vi "Anna_Auto.vi"() -> ()   [LabVIEW 2009]
panel:
  in  "notes":string
  out "Int duplex?":bool
  out "TACwinLoaded?":bool
  out "16btimage?":bool
  out "router":u8(ring) items=["sum", "0", "1", "2", "3", "4", "5", "6", "7", "8", "9", "10", "11", "12", "13", "14", "15"]
  out "plane":u32
  in  "router channel":u8
  in  "Value":cluster{"max":u32, "min":u32}
  out "what is done?":string
  in  "Folder Path":path
  out "what file?":path
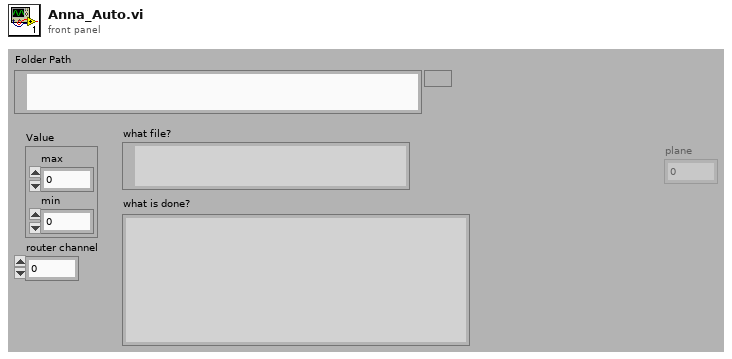
[diagram p1: front panel]
types:
  T1 = enum16{"Get", "Set", "Change", "ini", "clear", "draw", "draw false"}
  T2 = enum32{"existing file", "new file", "new or existing file", "existing dir", "new dir", "new or existing dir", "existing file (use LLBs)", "new file (use LLBs)", "new or existing file (use LLBs)", "new or existing file or directory (use LLBs)"}
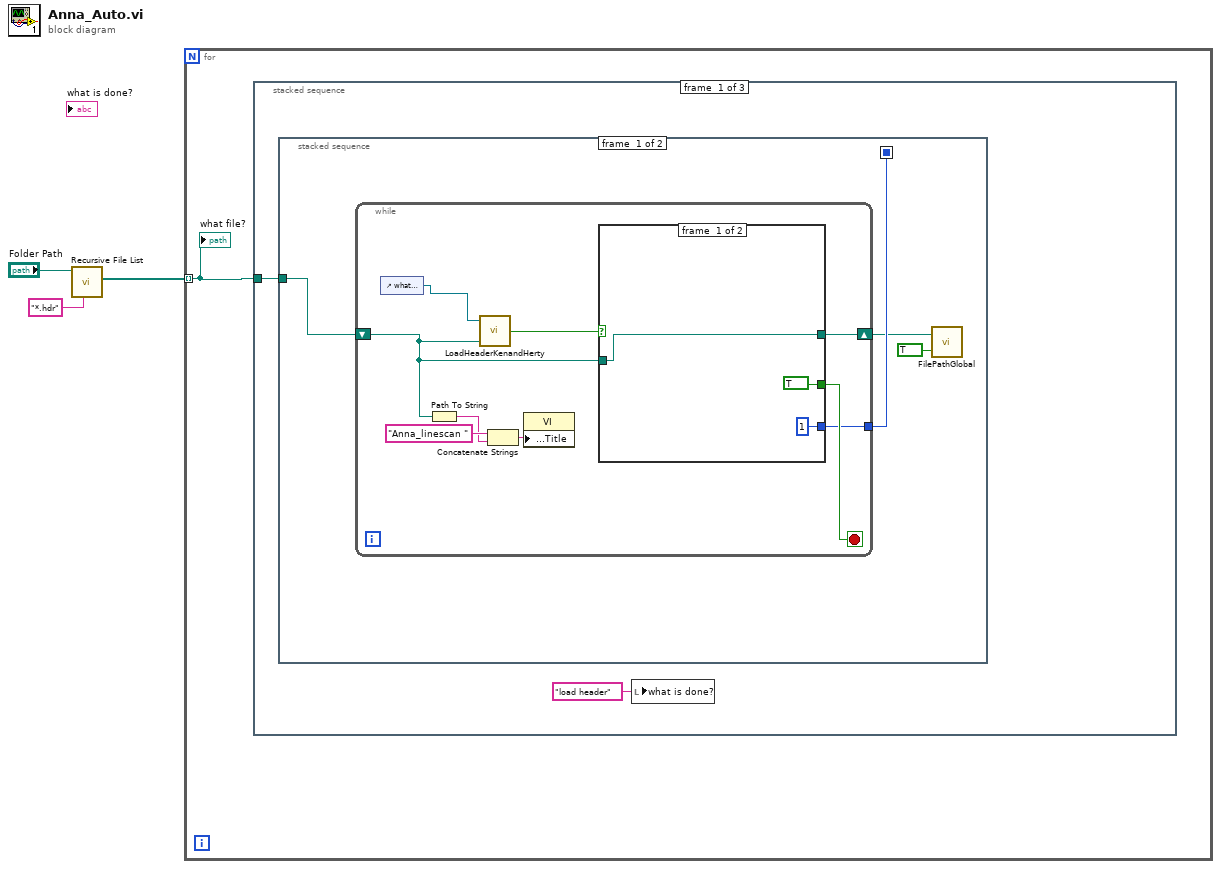
[diagram p0: block diagram]
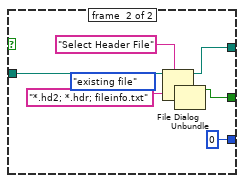
[diagram p2: hidden frame]
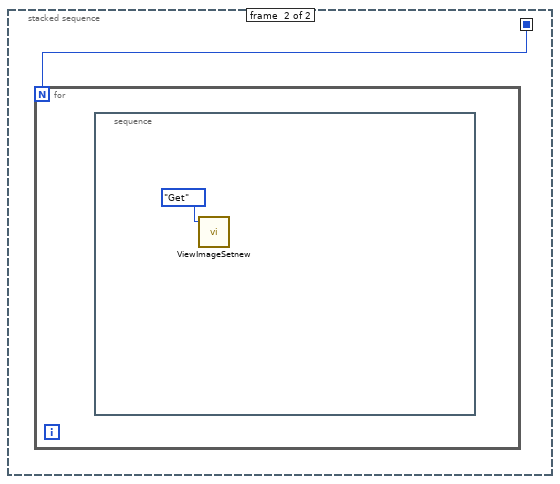
[diagram p3: hidden frame]
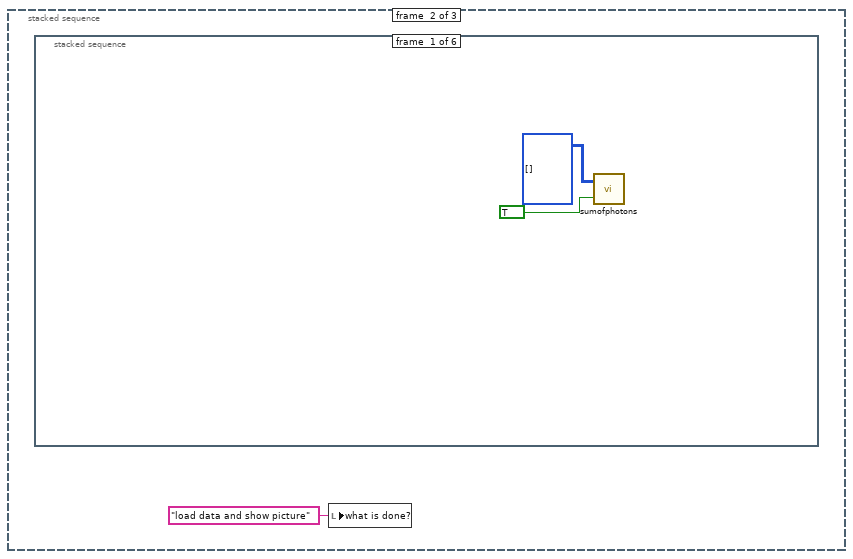
[diagram p4: hidden frame]
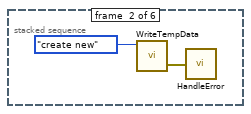
[diagram p5: hidden frame]
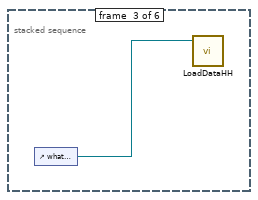
[diagram p6: hidden frame]
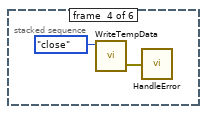
[diagram p7: hidden frame]
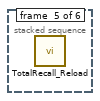
[diagram p8: hidden frame]
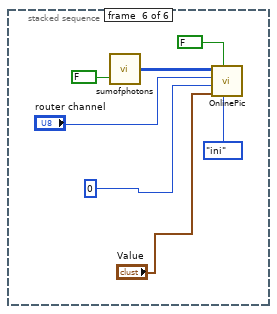
[diagram p9: hidden frame]
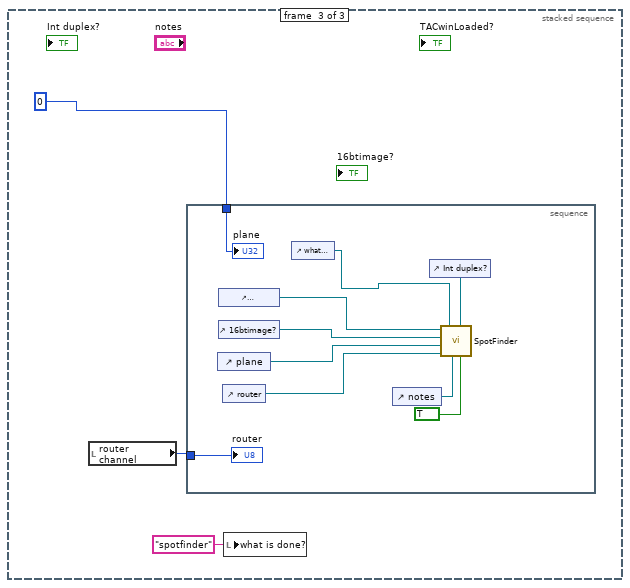
[diagram p10: hidden frame]
diagram:
  n1 = call <vilib>:"Recursive File List.vi"("pattern"="*.hdr", "Folder Path"="Folder Path") -> ("All Files in Dir"=w3:path[])  [unwired: 5 in, 4 out]
  n2 = for {
    tunnel: w3 -> [w4] mode=indexing
    n3 = stacked-sequence {
      tunnel: w4 -> [w6 _ _]
      frame #0 {
        n4 = stacked-sequence {
          seq-local: [w10 _] -> [_ w30]
          tunnel: w6 -> [w7 _]
          frame #0 {
            n5 = while {
              shift-right: [w13] -> w9
              shift-left: w7 -> [w14]
              tunnel: [w12] -> w10
              stop <- w15 stop-if-true
              n6 = control-ref of="what file?"() -> (w11:refnum<vi>)
              n7 = Path To String(path=w14) -> (string=w17:string)
              n8 = call "LoadHeaderKenandHerty.vi"("appended path"=w14, "reference"=w11) -> ("unsuccesful?"=w16:bool)  [unwired: 3 in]
              n9 = Concatenate Strings("Anna_linescan " ("string"), w17) -> (w19:string)
              n10 = property class="VI"("Front Panel Window:Title"=w19) -> ()  [unwired: 2 in, 2 out]
              n11 = case shown="False" w16 {
                tunnel: w14 -> [w20 w29]
                tunnel: [TRUE w25] -> w15
                tunnel: [w20 w27] -> w13
                tunnel: [1 0] -> w12
                frame #0 {
                }
                frame #1 {
                  (unwired) T2."existing file" ("select mode (2)")
                  n12 = File Dialog(6:"*.hd2; *.hdr; fileinfo.txt" ("pattern"), 7:"Select Header File" ("prompt"), 11:w29) -> (0:w23:errorcluster, 1:w25:bool, 3:w27:path)  [unwired: 4 in, 1 out]
                  n13 = Unbundle(w23) -> ()  [unwired: 3 out]
                }
              }
            }
            n14 = call "FilePathGlobal.vi"("Image Path"=w9, "set?"=TRUE) -> ()  [unwired: 3 out]
          }
          frame #1 {
            n15 = for {
              N: w30 -> [_]
              n16 = stacked-sequence {
                frame #0 {
                  n17 = call "ViewImageSetnew.vi"("action"=enum16{"Display", "change", "Get", "Set"}."Get" ("Enum")) -> ()  [unwired: 2 in, 1 out]
                }
              }
            }
          }
        }
        n18 = local write "what is done?"("load header" ("what is done?")) -> ()
      }
      frame #1 {
        n19 = stacked-sequence {
          frame #0 {
            n20 = call "sumofphotons.vi"("s"=TRUE, "sum of photons"=u32[][][][] []) -> ()  [unwired: 1 out]
          }
          frame #1 {
            n21 = call "WriteTempData.vi"("Enum"=enum16{"create new", "write", "close"}."create new") -> ("error out"=w35:errorcluster)  [unwired: 4 in, 1 out]
            n22 = call "HandleError.vi"("error in (no error)"=w35) -> ()
          }
          frame #2 {
            n23 = control-ref of="what file?"() -> (w37:refnum<vi>)
            n24 = call "LoadDataHH.vi"("Path"=w37) -> ()  [unwired: 2 in, 3 out]
          }
          frame #3 {
            n25 = call "WriteTempData.vi"("Enum"=enum16{"create new", "write", "close"}."close") -> ("error out"=w38:errorcluster)  [unwired: 4 in, 1 out]
            n26 = call "HandleError.vi"("error in (no error)"=w38) -> ()
          }
          frame #4 {
            n27 = call "TotalRecall_Reload.vi"() -> ()  [unwired: 4 in, 4 out]
          }
          frame #5 {
            n28 = call "sumofphotons.vi"("s"=FALSE) -> ("sum of photons out"=w44:u32[][][][])  [unwired: 1 in]
            n29 = call "OnlinePic.vi"("action"=T1."ini" ("Enum"), "RGB/False"=FALSE, "Threshold (max)"="Value", "plane"=u32 0, "router channel"="router channel", "Array"=w44) -> ()  [unwired: 1 in, 5 out]
          }
        }
        n30 = local write "what is done?"("load data and show picture" ("what is done?")) -> ()
      }
      frame #2 {
        n31 = local read "router channel"() -> (w47:u8)
        n32 = stacked-sequence {
          tunnel: u32 0 ("plane") -> [w52]
          tunnel: w47 -> [w51]
          frame #0 {
            n33 = control-ref of="plane"() -> (w56:refnum<vi>)
            n34 = control-ref of="TACwinLoaded?"() -> (w58:refnum<vi>)
            n35 = control-ref of="16btimage?"() -> (w57:refnum<vi>)
            n36 = control-ref of="router"() -> (w55:refnum<vi>)
            n37 = control-ref of="what file?"() -> (w53:refnum<vi>)
            n38 = control-ref of="notes"() -> (w54:refnum<vi>)
            n39 = control-ref of="Int duplex?"() -> (w59:refnum<vi>)
            n40 = call "SpotFinder.vi"("auto"=TRUE, "Int duplex?"=w59, "notes"=w54, "router 3"=w55, "plane 2"=w56, "Image Path"=w53, "16bit?"=w57, "TACwinLoaded?"=w58) -> ()  [unwired: 3 in]
            "plane" <- w52
            "router" <- w51
          }
        }
        n41 = local write "what is done?"("spotfinder" ("what is done?")) -> ()
      }
    }
    "what file?" <- w4
  }
